vi "Init Child.vi"(8 "error in (no error)":errorcluster, 11 "Git in":refnum<class "Git.lvclass">) -> (0 "error out":errorcluster, 3 "Git out":refnum<class "Git.lvclass">)   [LabVIEW 2020, in "Git.lvlib" / "Git.lvclass"]
uses:
  Git.lvclass
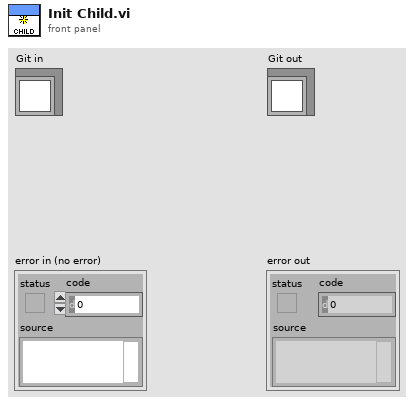
[diagram p1: front panel]
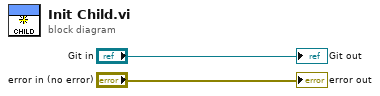
[diagram p0: block diagram]
diagram:
  "error out" <- "error in (no error)"
  "Git out" <- "Git in"
